vi "Conv_Heading_AngleRadians.vi"(10 "Heading":dbl) -> (2 "AngleRadians":dbl)   [LabVIEW 2019, in "Trajectory_Library.lvlib"]
doc: "This routine does nothing!"
uses:
  Trajectory_Library.lvlib
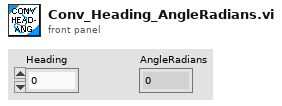
[diagram p1: front panel]
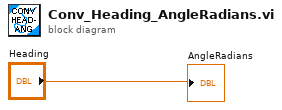
[diagram p0: block diagram]
diagram:
  "AngleRadians" <- "Heading"
